vi "ConfigureVelocityRegulator.vi"(0 "axis in":cluster{"keyHandle":u32, "nodeId":u16}={"keyHandle"=0, "nodeId"=1}, 7 "velocity gains":cluster{"p-Gain":u16, "i-Gain":u16}, 11 "error in (no error)":errorcluster) -> (4 "axis out":cluster{"keyHandle":u32, "nodeId":u16}={"keyHandle"=0, "nodeId"=1}, 15 "error out":errorcluster)   [LabVIEW 2019, in "maxonEPOS.lvlib"]
doc: "<B>ConfigureVelocityRegulator</B> writes the velocity regulation gain parameters to the device."
uses:
  Examples/maxonEPOS.lvlib
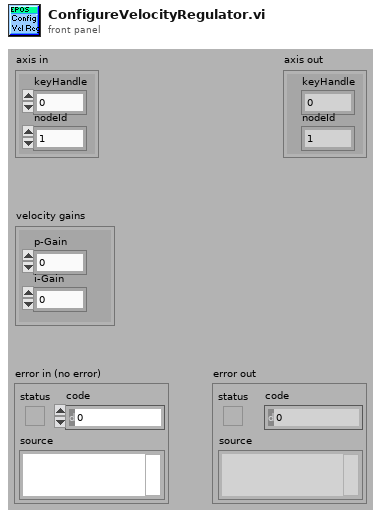
[diagram p1: front panel]
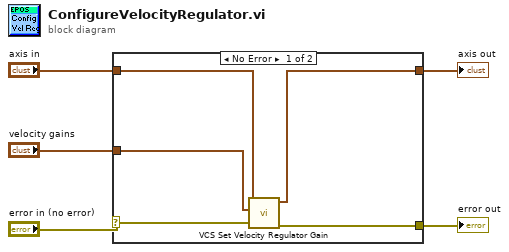
[diagram p0: block diagram]
diagram:
  n1 = case shown="No Error" "error in (no error)" {
    selector: "error in (no error)" -> [w9 w12]
    tunnel: [w8 w12] -> w4
    tunnel: [w7 w11] -> w3
    tunnel: "axis in" -> [w6 w11]
    tunnel: "velocity gains" -> [w10 _]
    frame No Error {
      n2 = call "VCS Set Velocity Regulator Gain.vi"("error in (no error)"=w9, "gains"=w10, "axis in"=w6) -> ("error out"=w8:errorcluster, "axis out"=w7:cluster{"keyHandle":u32, "nodeId":u16})  [unwired: 7 in]
    }
    frame Error {
    }
  }
  "error out" <- w4
  "axis out" <- w3
